vi "MQTT_ConnAck_Read.vi"(8 "error in (no error)":errorcluster, 11 "SSL_Connection":T1) -> (0 "error out":errorcluster, 1 "QoS Level":T3, 2 "Connection Status":T2=enum."Connection refused: not authorized", 3 "SSL_Connection":T1, 5 "MessageType":T4)   [LabVIEW 2018, in "AWS_IoT.lvlib"]
doc: "This VI processes the connection acknowledge message from the server.\n\n© 2015 - daq.io, LLC - Peter Adelhardt"
uses:
  AWS_IoT.lvlib
  Controls/MessageType.ctl
  Controls/QoS.ctl
  Controls/Connection_Return_Codes.ctl
  Controls/SSL_Connection.ctl
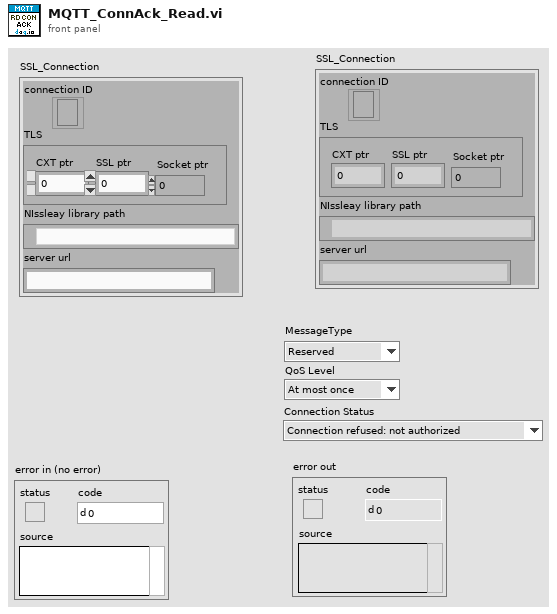
[diagram p1: front panel]
types:
  T1 = typedef "AWS_IoT.lvlib/SSL_Connection.ctl" = cluster{"connection ID":refnum<k5>, "TLS":cluster{"CXT ptr":i32, "SSL ptr":i32, "Socket ptr":i32}, "NIssleay library path":path, "server url":string}
  T2 = typedef "AWS_IoT.lvlib/Connection_Return_Codes.ctl" = enum16{"Connection accepted", "Connection refused: unacceptable protocol version", "Connection refused: identifier rejected", "Connection refused: Server unavailable", "Connection refused: bad user name or password", "Connection refused: not authorized"}
  T3 = typedef "AWS_IoT.lvlib/QoS.ctl" = enum8{"At most once", "At least once", "Exactly once", "Reserved"}
  T4 = typedef "AWS_IoT.lvlib/MessageType.ctl" = enum32{"Reserved", "CONNECT", "CONNACK", "PUBLISH", "PUBACK", "PUBREC", "PUBREL", "PUBCOMP", "SUBSCRIBE", "SUBACK", "UNSUBSCRIBE", "UNSUBACK", "PINGREQ", "PINGRESP", "DISCONNECT", "Reserved2"}
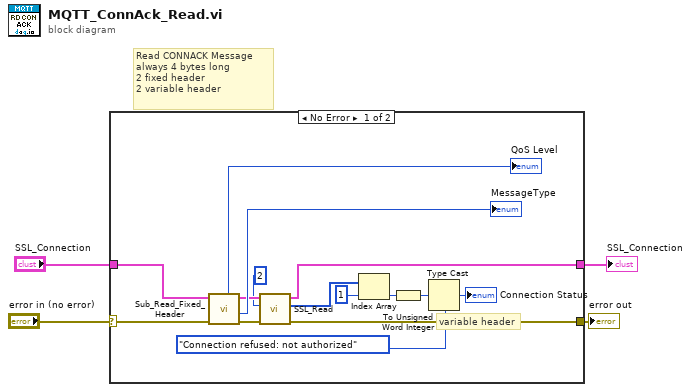
[diagram p0: block diagram]
diagram:
  # "Read CONNACK Message\nalways 4 bytes long\n2 fixed header\n2 variable header"
  n1 = case shown="No Error" "error in (no error)" {
    selector: "error in (no error)" -> [w17 w21]
    tunnel: [w11 w21] -> w3
    tunnel: "SSL_Connection" -> [w9 w20]
    tunnel: [w5 w20] -> w1
    frame No Error {
      # "variable header"
      n2 = call "Sub_Read_Fixed_Header.vi"("error in (no error)"=w17, "SSL_Connection"=w9) -> ("error out"=w12:errorcluster, "MessageType"=→"MessageType":T4, "SSL_Connection"=w8:T1, "QoS Level"=→"QoS Level":T3)  [unwired: 3 in, 3 out]
      n3 = call "SSL_Read.vi"("error in (no error)"=w12, "bytes to read"=2, "SSL_Connection"=w8) -> ("error out"=w11:errorcluster, "data out"=w7:u8[], "SSL_Connection"=w5:T1)  [unwired: 5 in, 1 out]
      n4 = Index Array(array=w7, index=1) -> (element=w19:u8)
      n5 = To Unsigned Word Integer(number=w19) -> (unsigned 16bit integer=w10:u16)
      n6 = Type Cast(type=Connection_Return_Codes."Connection refused: not authorized" ("Conn Return Code"), x=w10) -> (*(type *) &x=→"Connection Status":T2)
    }
    frame Error {
    }
  }
  "error out" <- w3
  "SSL_Connection" <- w1
